vi "Is CSM Module (Advanced).vi"(8 "error in (no error)":errorcluster, 10 "Active(F)":bool, 11 "VIRef":refnum<vi>) -> (0 "error out":errorcluster, 2 "Is CSM Module?":bool, 3 "VIRef(dup)":refnum<vi>)   [LabVIEW 2017, in "csm-tool-support.lvlib"]
uses:
  csm-tool-support.lvlib
panel:
  # "Connector Pane"
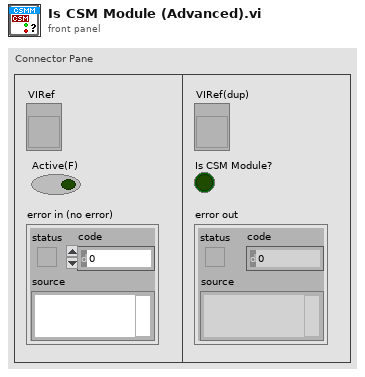
[diagram p1: front panel]
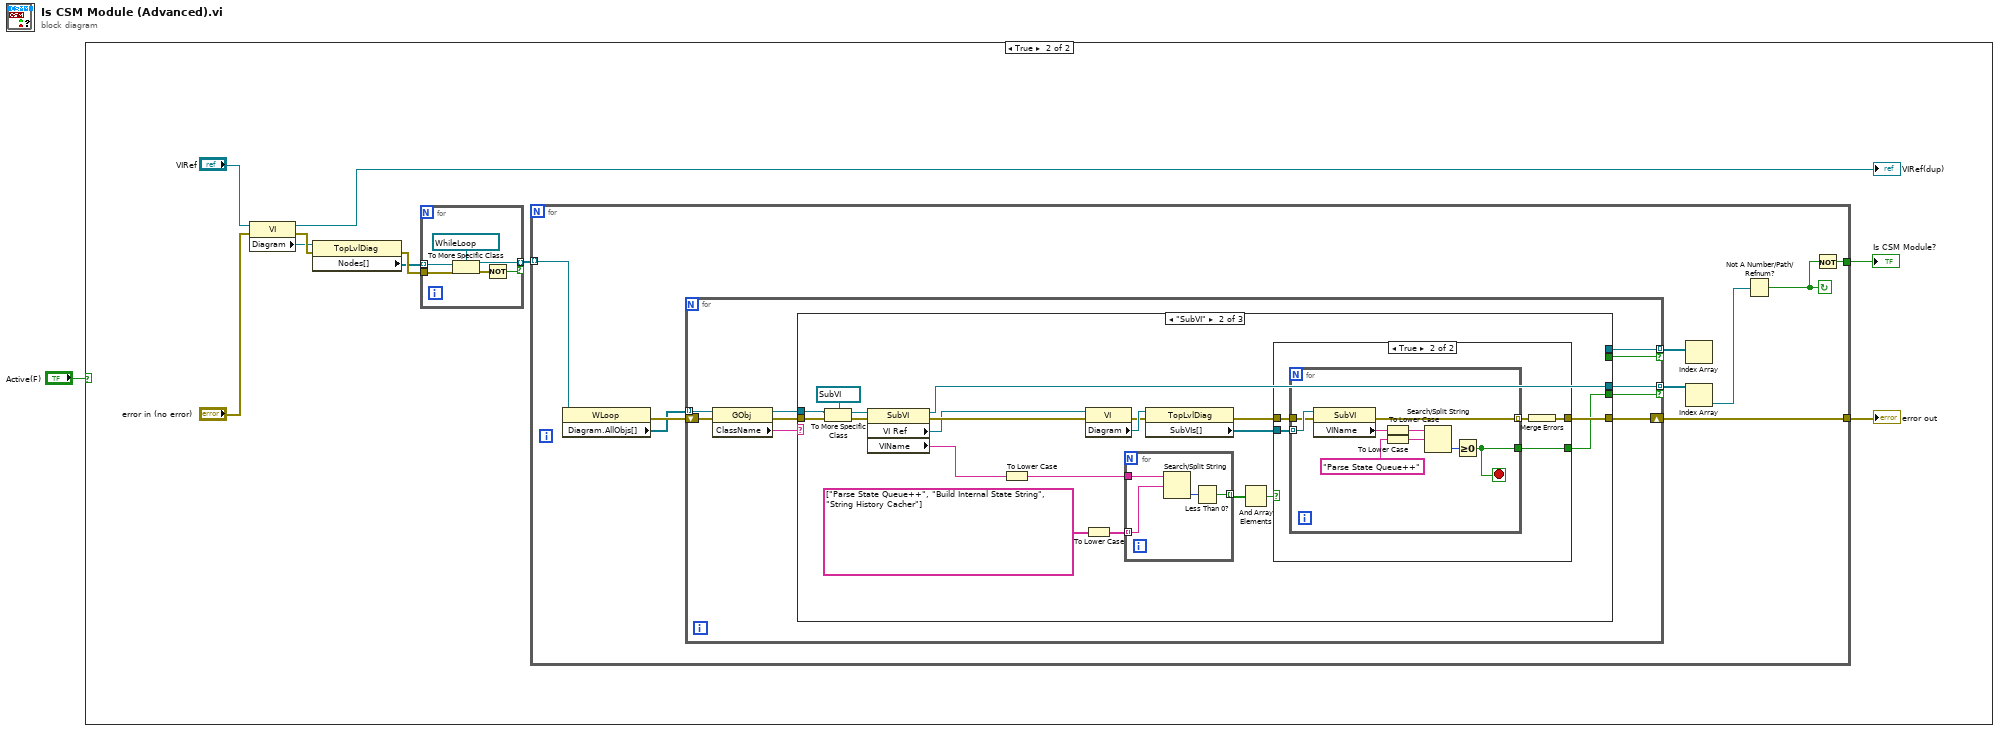
[diagram p0: block diagram]
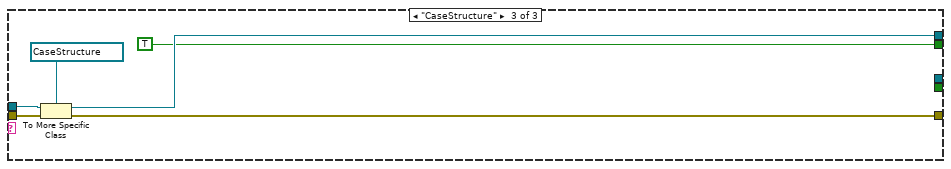
[diagram p5: hidden frame]
diagram:
  n1 = case shown="True" "Active(F)" {
    frame False {
    }
    frame True {
      n2 = property on="Property Node" class="VI"(reference="VIRef", error in="error in (no error)") -> (reference out=→"VIRef(dup)":refnum<vi>, error out=w9:errorcluster, "Diagram"=w6:refnum<vi>)
      n3 = property on="Property Node" class="TopLvlDiag"(reference=w6, error in=w9) -> (error out=w8:errorcluster, "Nodes[]"=w7:refnum<vi>[])  [unwired: 1 out]
      n4 = for {
        tunnel: w7 -> [w81] mode=indexing
        tunnel: [w79] -> w5 mode=indexing if=w77
        tunnel: w8 -> [w80]
        n5 = To More Specific Class(target class=refnum<vi> refnum ("WLoop Refnum"), reference=w81, error in=w80) -> (specific class reference=w79:refnum<vi>, error out=w78:errorcluster)
        n6 = Not(x=w78) -> (.not. x?=w77:bool)
      }
      n7 = for {
        tunnel: w5 -> [w19] mode=indexing
        tunnel: [w20] -> w4
        tunnel: [w16] -> w2
        stop <- w17 continue-if-true
        n8 = property on="Property Node" class="WLoop"(reference=w19) -> (error out=w13:errorcluster, "Diagram.AllObjs[]"=w12:refnum<vi>[])  [unwired: 1 in, 1 out]
        n9 = for {
          tunnel: w12 -> [w30] mode=indexing
          shift-right: [w25] -> w20
          shift-left: w13 -> [w26]
          tunnel: [w24] -> w15 mode=indexing if=w21
          tunnel: [w23] -> w14 mode=indexing if=w22
          n10 = property class="GObj"(reference=w30, error in=w26) -> (reference out=w28:refnum<vi>, error out=w27:errorcluster, "ClassName"=w29:string)
          n11 = case shown="\"SubVI\"" w29 {
            tunnel: w28 -> [_ w50 w75]
            tunnel: w27 -> [w31 w49 w74]
            tunnel: [w31 w33 w73] -> w25
            tunnel: [_ w43 _] -> w24
            tunnel: [_ _ w72] -> w23
            tunnel: [_ _ TRUE] -> w22
            tunnel: [_ w32 _] -> w21
            frame Default {
            }
            frame "SubVI" {
              n12 = To More Specific Class(target class=refnum<vi> refnum ("SubVI Refnum"), reference=w50, error in=w49) -> (specific class reference=w48:refnum<vi>, error out=w47:errorcluster)
              n13 = property class="SubVI"(reference=w48, error in=w47) -> (reference out=w43:refnum<vi>, error out=w44:errorcluster, "VI Ref"=w42:refnum<vi>, "VIName"=w39:string)
              n14 = To Lower Case(string=w39) -> (all lower case string=w38:string)
              n15 = property class="VI"(reference=w42, error in=w44) -> (error out=w40:errorcluster, "Diagram"=w41:refnum<vi>)  [unwired: 1 out]
              n16 = To Lower Case(string=string[] ["Parse State Queue++", "Build Internal State String", "String History Cacher"] ("VI Name")) -> (all lower case string=w45:string[])
              n17 = for {
                tunnel: w45 -> [w68] mode=indexing
                tunnel: w38 -> [w69]
                tunnel: [w67] -> w37 mode=indexing
                n18 = Search/Split String(string=w69, search string/char (-)=w68) -> (offset of match=w70:i32)  [unwired: 1 in, 2 out]
                n19 = Less Than 0?(x=w70) -> (x < 0?=w67:bool)
              }
              n20 = property class="TopLvlDiag"(reference=w41, error in=w40) -> (error out=w35:errorcluster, "SubVIs[]"=w36:refnum<vi>[])  [unwired: 1 out]
              n21 = And Array Elements(Boolean array=w37) -> (logical AND=w34:bool)
              n22 = case shown="True" w34 {
                tunnel: w36 -> [_ w57]
                tunnel: w35 -> [w52 w56]
                tunnel: [w52 w54] -> w33
                tunnel: [_ w53] -> w32
                frame False {
                }
                frame True {
                  n23 = for {
                    tunnel: w57 -> [w66] mode=indexing
                    tunnel: w56 -> [w65]
                    tunnel: [w59] -> w53
                    tunnel: [w58] -> w55 mode=indexing
                    stop <- w59 stop-if-true
                    n24 = property class="SubVI"(reference=w66, error in=w65) -> (error out=w58:errorcluster, "VIName"=w64:string)  [unwired: 1 out]
                    n25 = To Lower Case(string=w64) -> (all lower case string=w62:string)
                    n26 = To Lower Case(string="Parse State Queue++" ("VI Name")) -> (all lower case string=w60:string)
                    n27 = Search/Split String(string=w62, search string/char (-)=w60) -> (offset of match=w63:i32)  [unwired: 1 in, 2 out]
                    n28 = Greater Or Equal To 0?(x=w63) -> (x >= 0?=w59:bool)
                  }
                  n29 = Merge Errors(w55) -> (w54:errorcluster)
                }
              }
            }
            frame "CaseStructure" {
              n30 = To More Specific Class(target class=refnum<vi> refnum ("CaseSel Refnum"), reference=w75, error in=w74) -> (specific class reference=w72:refnum<vi>, error out=w73:errorcluster)
            }
          }
        }
        n31 = Index Array(array=w14) -> ()  [unwired: 1 in, 1 out]
        n32 = Index Array(array=w15) -> (element=w18:refnum<vi>)  [unwired: 1 in]
        n33 = Not A Number/Path/Refnum?(number/path/refnum=w18) -> (NaN/Path/Refnum?=w17:bool)
        n34 = Not(x=w17) -> (.not. x?=w16:bool)
      }
      "error out" <- w4
      "Is CSM Module?" <- w2
    }
  }
